vi "Window-Functional data editor - variable patch.vi"(9 "Experiment Path":path=path "D:/Microscope data/Sameer/2019-10-16/191016_19_21_07 FunctAcq", 11 "Standalone viewer?":bool=TRUE) -> ()   [LabVIEW 2020]
uses:
  User Interface/Visualisation/Timelapse Viewer/Typedefs/Custom slider-vertical.ctl
  User Interface/Visualisation/Timelapse Viewer/Typedefs/Colour.ctl
  User Interface/Visualisation/Timelapse Viewer/Typedefs/Channel to load.ctl
  User Interface/Visualisation/Timelapse Viewer/Typedefs/Time series viewer refs.ctl
  User Interface/Visualisation/Timelapse Viewer/Typedefs/Speed Viewer States enum.ctl
  <vilib>/Utility/miscctls.llb/LVPointTypeDef.ctl
  <vilib>/vision/Image Controls.llb/IMAQ Image.ctl
  Typedefs/HW config states enum.ctl
  User Interface/Visualisation/Functional Imaging Viewer/Typedefs/Get-Set-Clear Control.ctl
  User Interface/Visualisation/Timelapse Viewer/Typedefs/Select Play-Stop button to show.ctl
  <vilib>/Utility/error.llb/DialogType.ctl
  User Interface/Visualisation/Timelapse Viewer/Cam video sync/Typedefs/Cam videos cluster.ctl
  User Interface/Visualisation/Timelapse Viewer/Globals/gl_Time series viewer globals.vi
  Global Variables/General Globals.vi
  Typedefs/Save-Load enum.ctl
panel:
  in  "Image Scrollbar":i32(c297)
  out "VL Image Array":T1[](array[plugin-control])
  in  "Channel to load":T2
  in  "Number of rows to generate":i32=3 format="%.0f rows"
  in  "Source number of frames":T3(ring)=enum."As many as the number of cycles"
  out "Slider at frame #":i32 format="Cycle %.0f"
  in  "Scrollbar":i32(c297)
  in  "Back":bool
  in  "Play":bool
  in  "Stop":bool
  in  "Tab Control":enum32{"Camera videos", "Speed data"}(tab)
  out "Cams":T4 {"Vid4 Rel time (ms)" format="%.0f ms"; "Vid3 Rel time (ms)" format="%.0f ms"; "Vid2 Rel time (ms)" format="%.0f ms"; "Vid1 Rel time (ms)" format="%.0f ms"}
  out "Actual number \nof speed points":i32 format="Actual of speed points: %.0f"
  out "Speed Data":string[][](array[string])
  out "Expected speed values":dbl format="Expected speed points: %#_g"
  out "Original frame rate (fps)":dbl format="Original frame rate: %#.1f (fps)"
  out "Frame rate set (fps)":dbl format="Frame rate set: %#.1f (fps)"
  out "Actual frame rate (fps)":dbl format="Actual frame rate: %#.1f (fps)"
  out "AVI Mode ind":string="AVI mode:"
  out "Video length info":string="Duration: 00h 00m 00s, 0 frames"
  out "Export images":bool
  out "Export snippet":bool
  in  "Extraction Cursors":cluster{i32, i32}(slide)={1, 5594} scale=1.0..1109.0
  out "Export vid":bool
  out "Stop (ind)":bool
  in  "Intensity":T5={0.0, 4095.0} scale=0.0..4095.0
  in  "Colour":T6
  out "Speed Graph":dbl[](graph) caption="Speed Chart"
  out "Image":T1(plugin-control)
  # "Date                         Time                  Time stamp           Speed (rpm)          Angle (deg)"
  # "Timelapse Info"
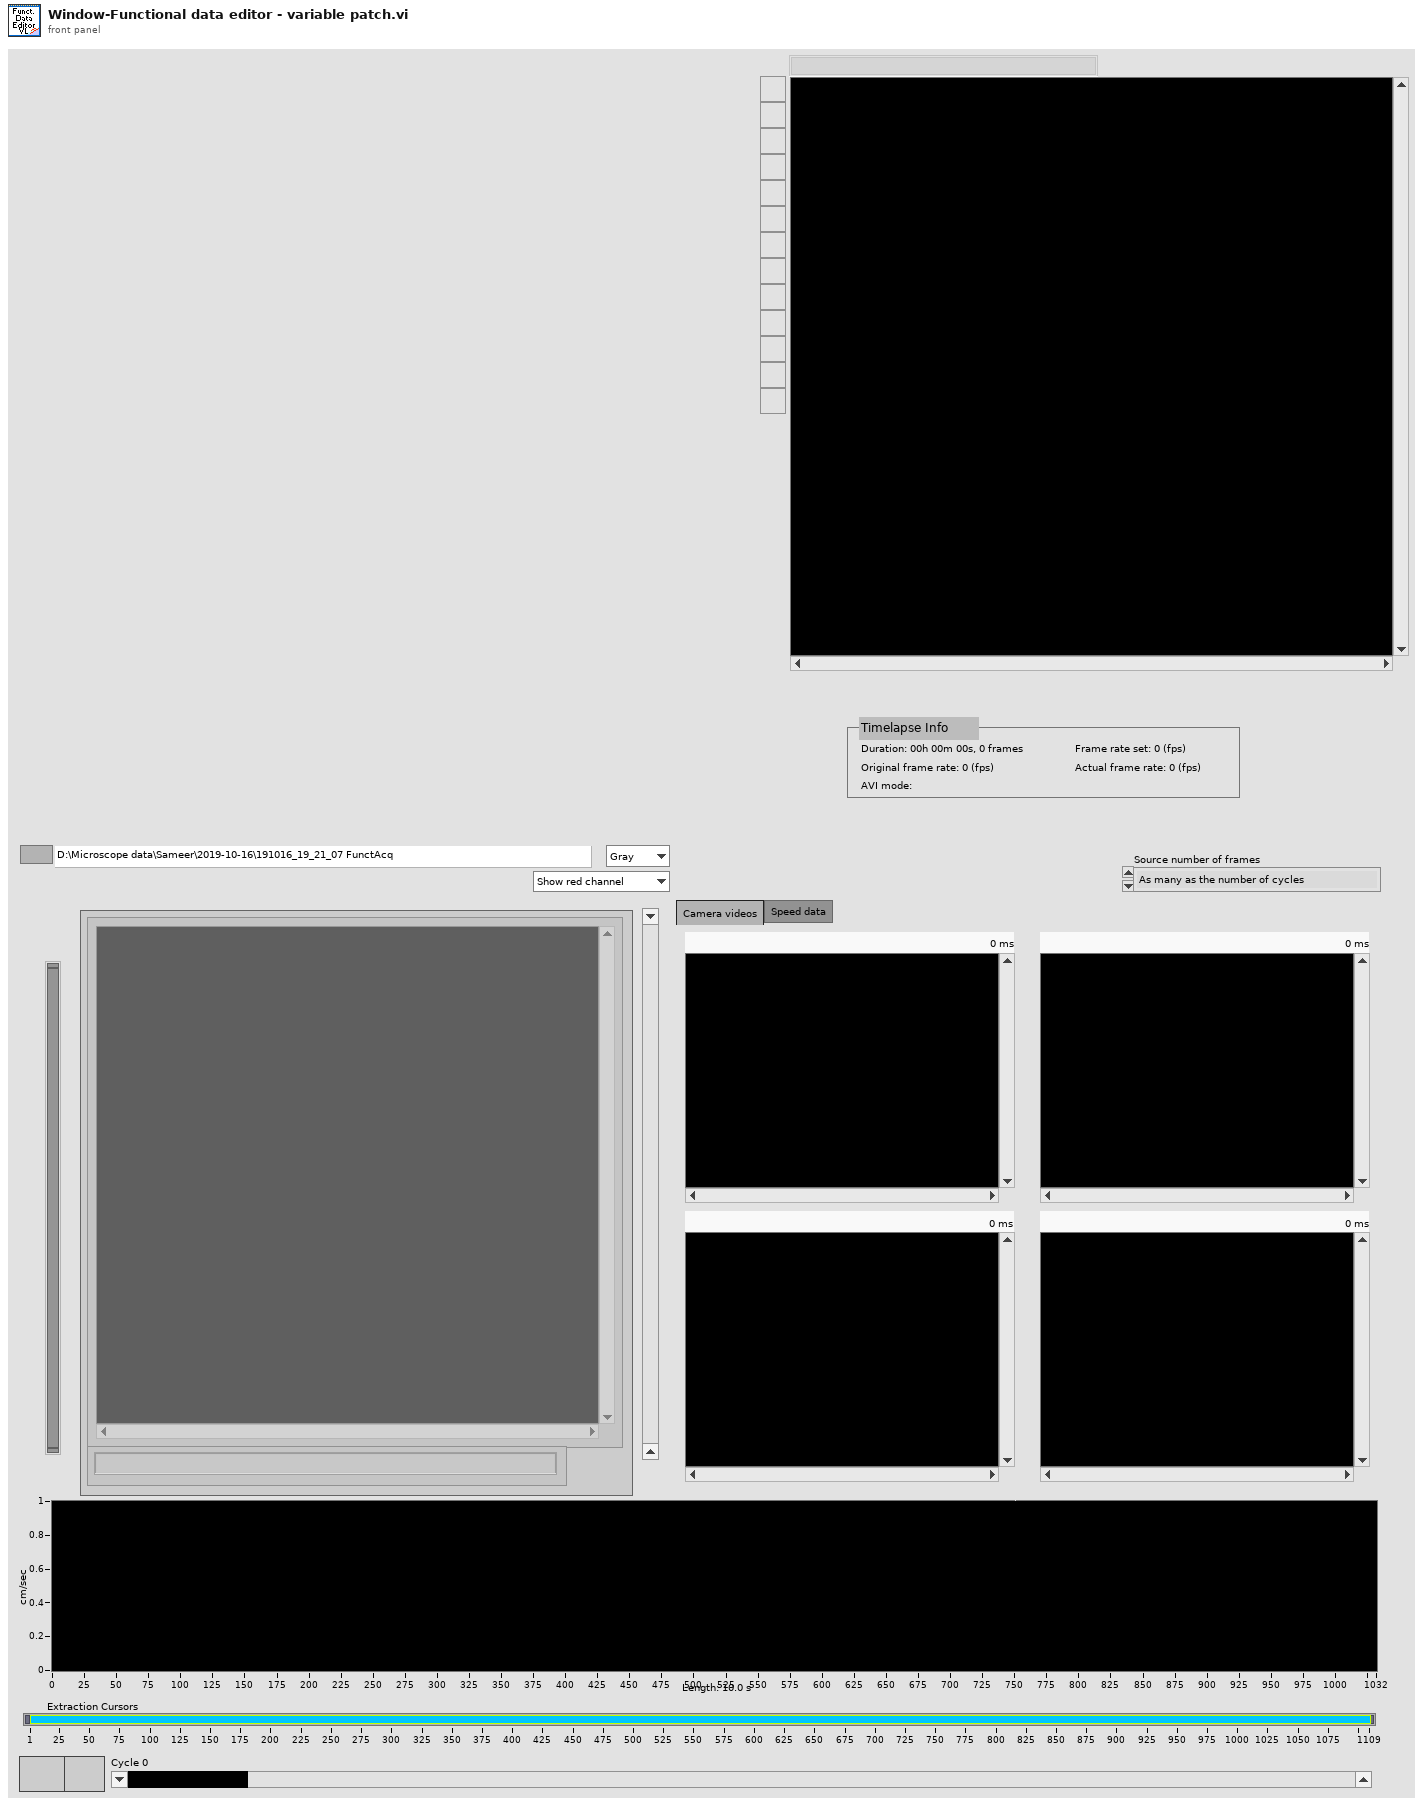
[diagram p1: front panel]
types:
  T1 = typedef "IMAQ Image.ctl" = refnum<image>
  T2 = typedef "Channel to load.ctl" = enum16{"Show red channel", "Show green channel", "Show both channels"}
  T3 = enum16{"As many as the frames in the video with the fewest frames", "As many as the number of cycles"}
  T4 = cluster{"Vid 1":T1, "Vid 2":T1, "Vid 3":T1, "Vid 4":T1, "Vid1 Rel time (ms)":u32, "Vid2 Rel time (ms)":u32, "Vid3 Rel time (ms)":u32, "Vid4 Rel time (ms)":u32}
  T5 = typedef "Custom slider-vertical.ctl" = cluster{dbl, dbl}
  T6 = typedef "Colour.ctl" = enum16{"Gray", "Red", "Green", "Mixed"}
  T7 = typedef "Time series viewer refs.ctl" = cluster{"This VI":refnum<vi>, "Image control":refnum<vi>, "AVI Mode ind":refnum<vi>, "Play":refnum<vi>, "Stop":refnum<vi>, "Back":refnum<vi>, "Scrollbar":refnum<vi>, "Video length info":refnum<vi>, "Expected speed values":refnum<vi>, "Intensity":refnum<vi>, "Path":refnum<vi>, "Selection sliders":refnum<vi>, "Speed Graph ref":refnum<vi>, "Frame rate set (fps)":refnum<vi>, "Number of rows to generate":refnum<vi>, "VL Image Array":refnum<vi>, "Image Scrollbar":refnum<vi>, "Channel to load":refnum<vi>, "Colour":refnum<vi>}
  T8 = enum16{"None", "Release queue", "Obtain queue", "Enqueue", "Get status", "Set status"}
  T9 = typedef "LVPointTypeDef.ctl" = cluster{"Horizontal":i16, "Vertical":i16}
  T10 = typedef "Speed Viewer States enum.ctl" = enum16{"Idle", "Initialise", "Playback", "Scroll bar event", "Speed cursor event", "Back to start", "Exit"}
  T11 = typedef "Save-Load enum.ctl" = enum16{"Save to file", "Load from file", "Compare from file", "Save Backup"}
  T12 = typedef "HW config states enum.ctl" = enum16{"Load from file", "Save to file", "Save backup", "Write all", "Read all", "Write XY stage settings", "Write DAQ FPGA settings", "Write Control FPGA settings", "Write Phys Channels", "Write System Config", "Write HW Config", "Save System Config", "Save HW Config", "Clear", "Compare from file"}
  T13 = typedef "Image Type" = u32
  T14 = typedef "Custom slider-horisontal.ctl" = cluster{dbl, dbl}
  T15 = typedef "Cam videos cluster.ctl" = cluster{"Vid 1":T1, "Vid 2":T1, "Vid 3":T1, "Vid 4":T1, "Vid1 Rel time (ms)":u32, "Vid2 Rel time (ms)":u32, "Vid3 Rel time (ms)":u32, "Vid4 Rel time (ms)":u32}
  T16 = typedef "Get-Set-Clear Control.ctl" = enum16{"Get", "Set", "Clear"}
  T17 = typedef "Select Play-Stop button to show.ctl" = enum16{"Show Play button", "Show Stop button"}
  T18 = typedef "DialogType.ctl" = u16
  T19 = typedef "Hardware Configuration settings.ctl" = cluster{"Dev. PC":bool, "Swap XY on stage":bool, "No of AOD":u8, "MC Supported":bool, "Axial MC":bool, "Computer MAC address":string, "Externalise Triggers":bool, "Trigger HW config":T20, "DAQmx Chan":T21, "XYZ Stage Control Config":T22, "XY stage available":bool, "XY Comms Config Cluster":T23, "Y stage available":bool, "Y Comms Config Cluster":T23, "Z stage available":bool, "Z Comms Config Cluster ":T23, "Encoder available":bool, "Encoder":T25, "VidRec available":bool, "Cam VidRec":T26, "Laser Power Control HW config":T27, "Laser 1 available":bool, "Laser 1 config cluster":T28, "Prechirper 1 available":bool, "Prechirper 1 config cluster":T29, "Control system.FPGA available?":bool, "Control Sys. HW config":T30, "DAQ FPGA HW Config":T31, "PMT Control Voltage Limits":T35}
  T20 = typedef "Triggers HW config.ctl" = cluster{"Available Device List":i32, "Device Address":string}
  T21 = typedef "DAQmx physical channels cluster.ctl" = cluster{"Pockels AO":tag, "Hard shutter AO":tag, "PMT AOs":tag, "Galvo AOs":tag, "Power meter AI":tag}
  T22 = typedef "XYZControlConfig.ctl" = enum16{"None", "XYZ", "XY-Z", "X-Y-Z", "Z"}
  T23 = typedef "Peripherals comms config cluster.ctl" = cluster{"Name":string, "Device Address":string, "Port ":u16, "Baudrate":i32, "Comms Type":T24}
  T24 = typedef "Comms Type.ctl" = enum16{"GPIB-IEEE488", "Serial-RS232", "Serial-RS485", "Serial-RS422", "Serial-USB", "Ethernet-TCP/IP", "Ethernet-UDP"}
  T25 = typedef "Encoder config cluster.ctl" = cluster{"IP address":string, "Port":u16, "Wheel radius (cm)":dbl, "Encoder Trigger":tag}
  T26 = typedef "Cam VidRec HW config setup cluster.ctl" = cluster{"DO flag-Video record":tag, "DO flag-Trial start":tag}
  T27 = typedef "Laser Power Control HW config.ctl" = cluster{"Laser Power Control":string, "Laser Power Modulation Control":enum16{"NI", "FPGA"}}
  T28 = typedef "Laser 1 config cluster.ctl" = cluster{"COM port":refnum<visa-resource-name>, "Baud Rate":i32, "Type":string}
  T29 = typedef "PreChirper 1 config cluster.ctl" = cluster{"Type":string, "Baud Rate":i32, "COM port":refnum<visa-resource-name>}
  T30 = typedef "Control Sys HW config cluster.ctl" = cluster{"Control system.FPGA Type":enum16{"Virtex 5", "Virtex 7"}, "Control system.Network adapter name":string, "Control system.MAC address":string, "Control system.Ethernet Port":u32, "Control system.Ethernet Port Opened":bool}
  T31 = typedef "DAQ FPGA HW config cluster.ctl" = cluster{"FGPA Ref":T32, "Target":T33, "input card type":T34}
  T32 = typedef "FPGA Ref.ctl" = refnum<k20>
  T33 = typedef "nirio_resource_hc.ctl" = tag
  T34 = typedef "FPGA input type AC-DC.ctl" = enum16{"AC Card", "DC Card"}
  T35 = typedef "PMT Control Voltage limits.ctl" = cluster{"Lower Limit":dbl, "Upper Limit":dbl}
  T36 = cluster{"Start Frame No":i32, "End Frame No":i32}
  T37 = typedef "IMAQ AVI2 Refnum.ctl" = refnum<k20>
  T38 = cluster{"# of frames to export":i32, "Initial frame's owning file":T37, "8-bit AVI file path":path, "Cursors location":cluster{"Number of first frame":i32, "Number of last frame":i32}}
  T39 = enum32{"Invalid", "Standard", "Closed", "Hidden", "Minimized", "Maximized"}
  T40 = typedef "Speed graph behaviour enum.ctl" = enum16{"Scrolling data", "Scrolling cursor"}
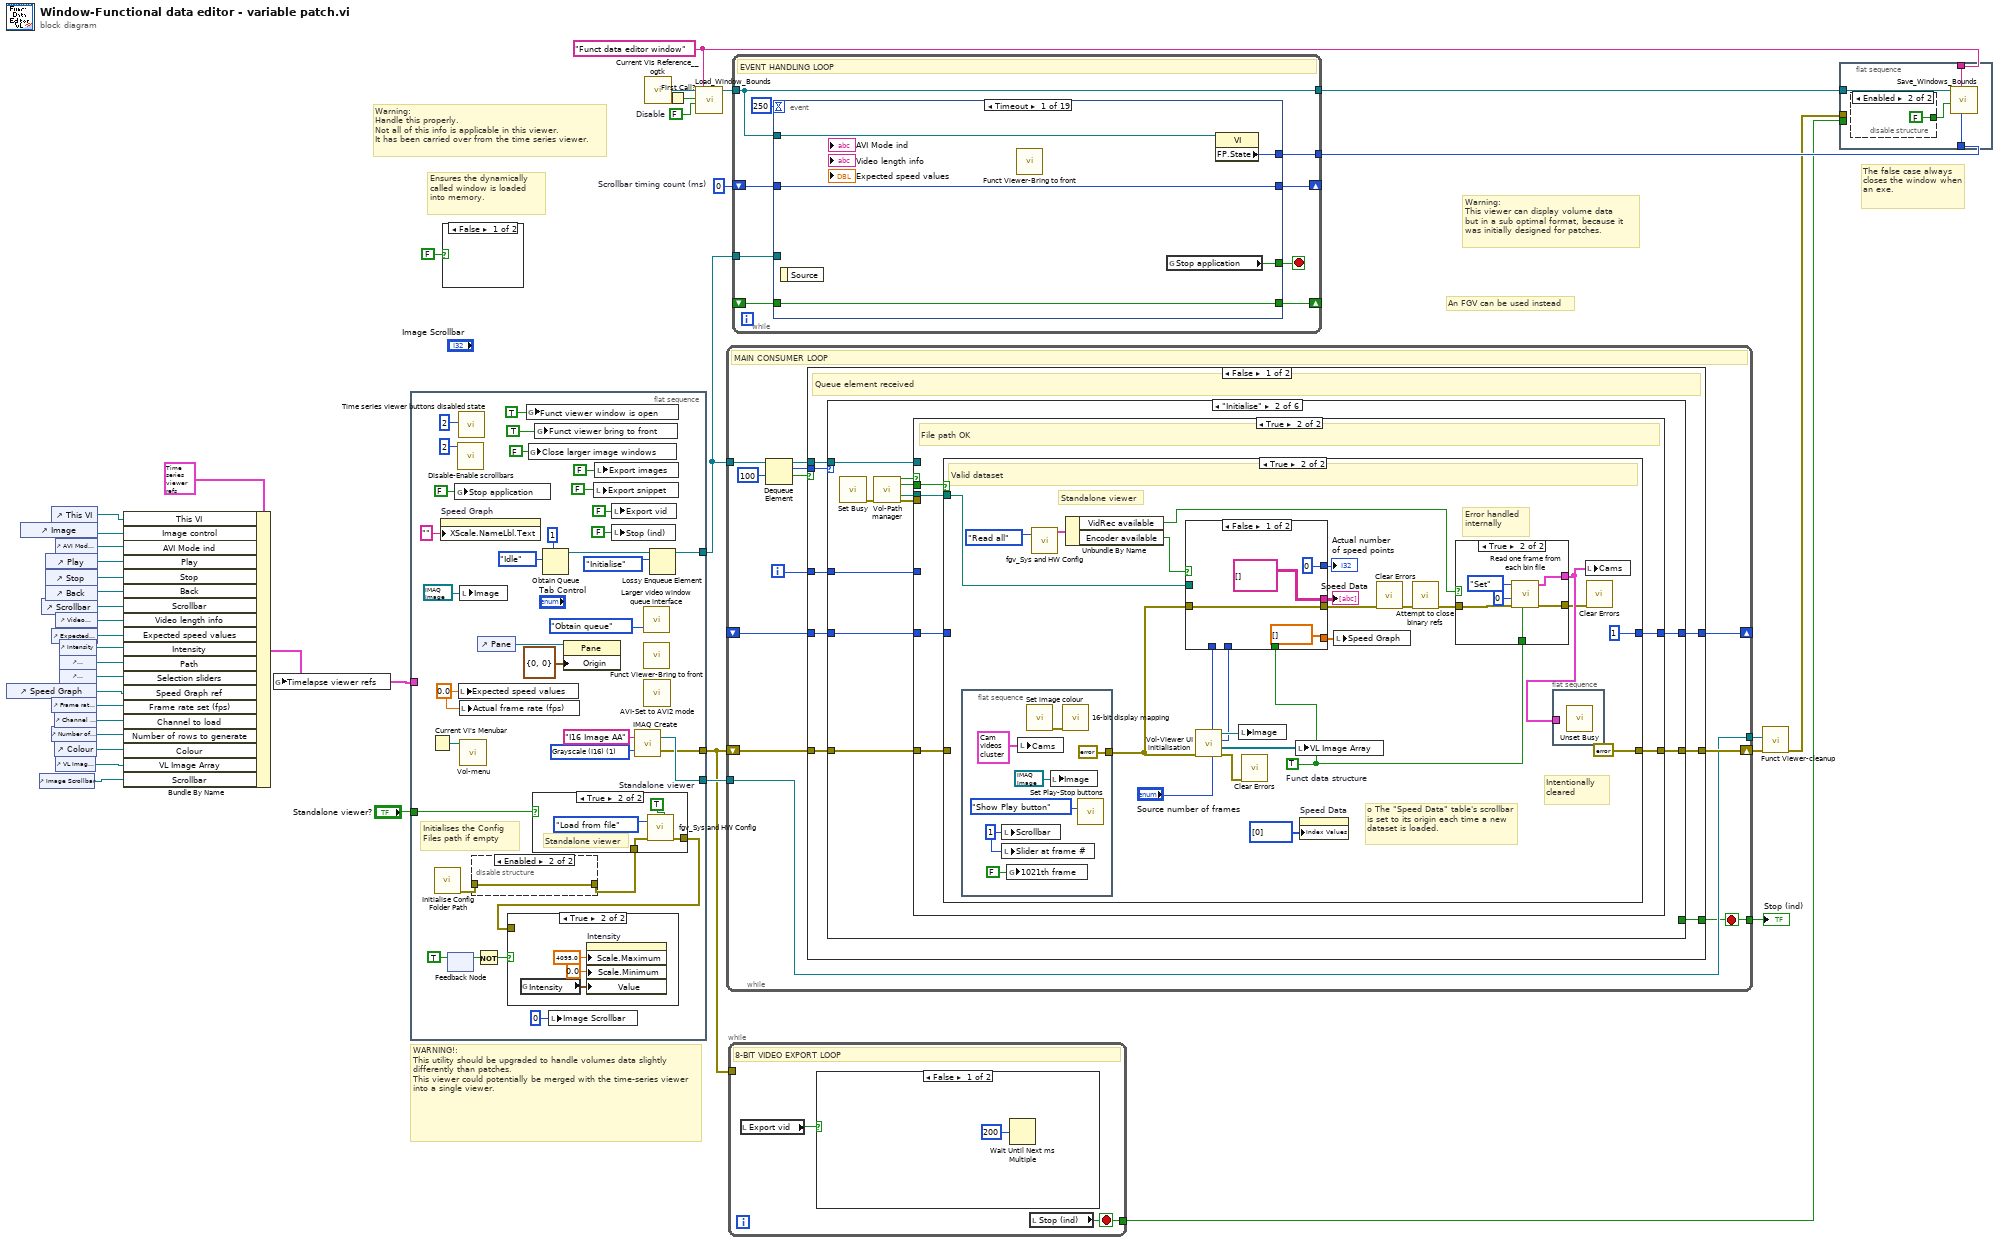
[diagram p0: block diagram]
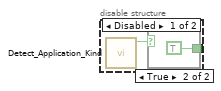
[diagram p2: hidden frame]
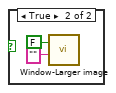
[diagram p4: hidden frame]
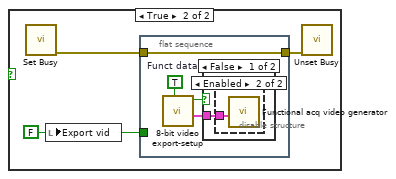
[diagram p5: hidden frame]
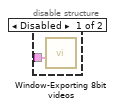
[diagram p6: hidden frame]
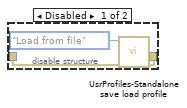
[diagram p8: hidden frame]
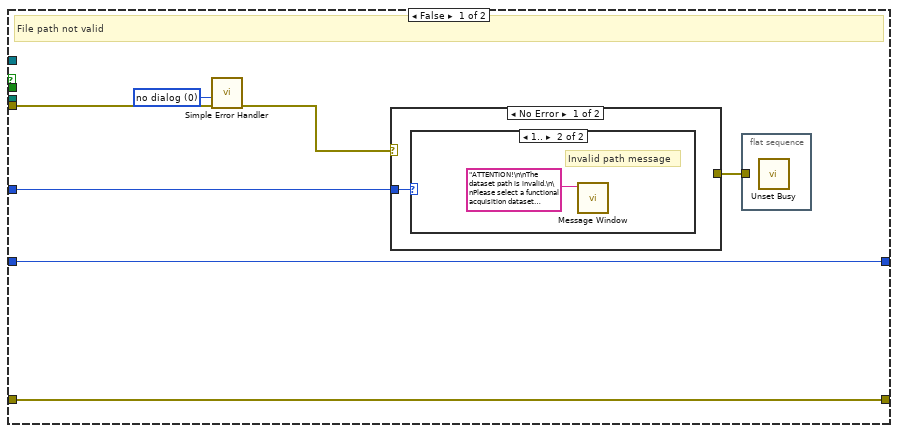
[diagram p12: hidden frame]
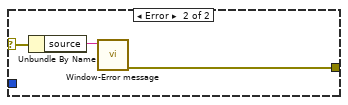
[diagram p14: hidden frame]
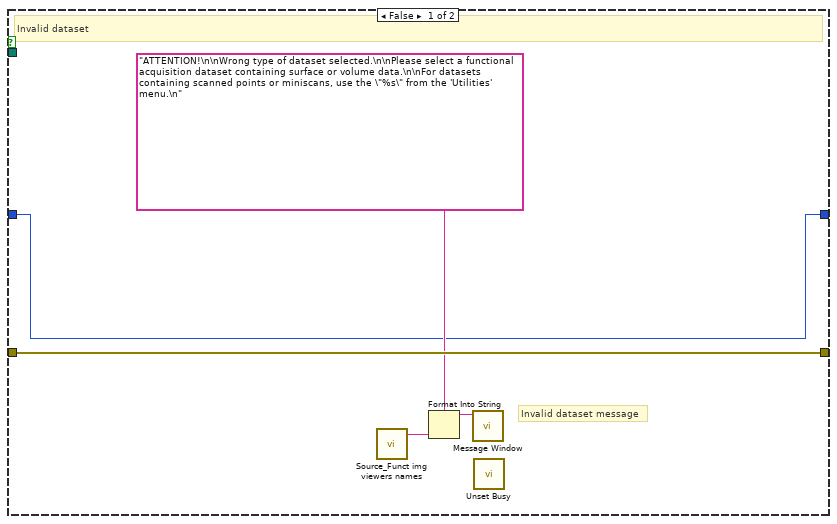
[diagram p15: hidden frame]
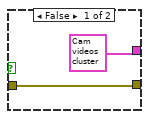
[diagram p16: hidden frame]
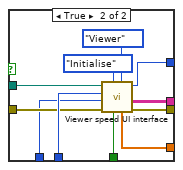
[diagram p17: hidden frame]
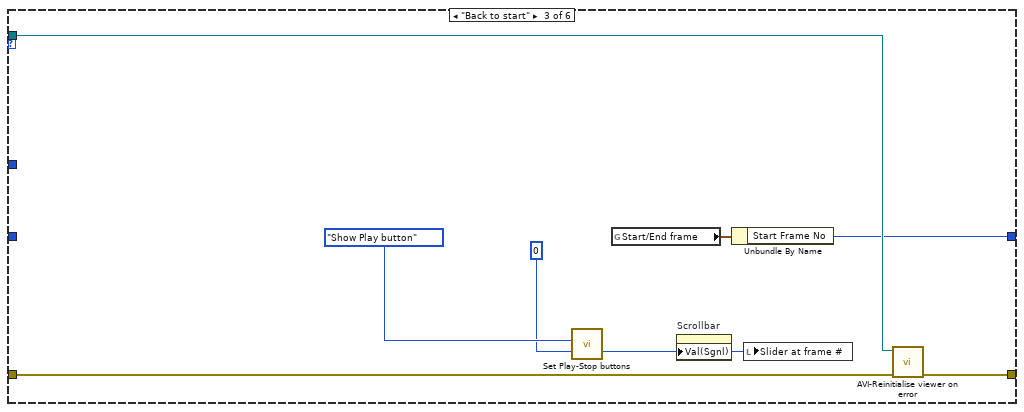
[diagram p18: hidden frame]
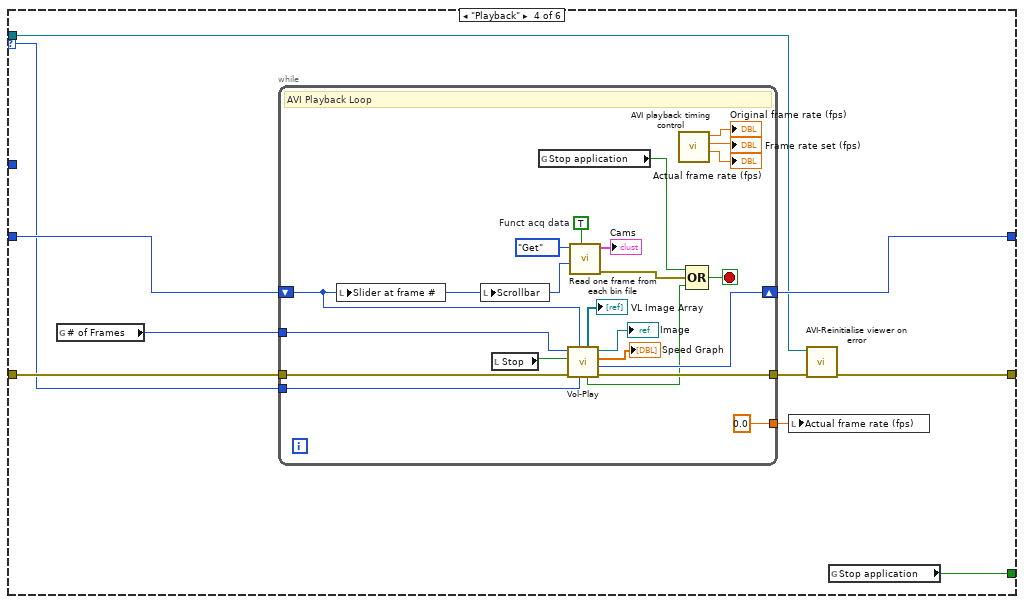
[diagram p19: hidden frame]
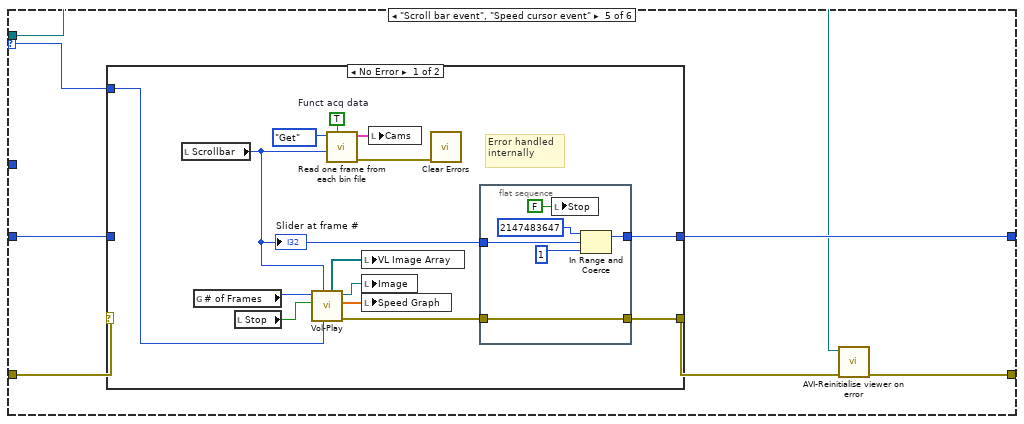
[diagram p20: hidden frame]
diagram:
  w17 = FALSE  # Disable
  w16 = "Funct data editor window" ("Window Name (i.e. Key)")
  w26 = u32 0  # Scrollbar timing count (ms)
  # "Warning:\nThis viewer can display volume data\nbut in a sub optimal format, because it\nwas initially designed for patches."
  # "Warning:\nHandle this properly.\nNot all of this info is applicable in this viewer.\nIt has been carried over from the time series viewer."
  # "WARNING!:\nThis utility should be upgraded to handle volumes data slightly differently than patches.\nThis viewer could potentially be merged with the time-series viewer into a single viewer."
  # "The false case always closes the window when an exe."
  # "Ensures the dynamically called window is loaded into memory."
  # "An FGV can be used instead"
  n1 = control-ref of="Speed Graph"() -> (w21:refnum<vi>)
  n2 = control-ref of="Image"() -> (w6:refnum<vi>)
  n3 = control-ref of="Image Scrollbar"() -> (w3:refnum<vi>)
  n4 = control-ref of="Scrollbar"() -> (w30:refnum<vi>)
  n5 = control-ref of="Play"() -> (w33:refnum<vi>)
  n6 = control-ref of="Stop"() -> (w32:refnum<vi>)
  n7 = control-ref of="Back"() -> (w31:refnum<vi>)
  n8 = control-ref of="Frame rate set (fps)"() -> (w10:refnum<vi>)
  n9 = control-ref of="Number of rows to generate"() -> (w8:refnum<vi>)
  n10 = control-ref of="This VI"() -> (w24:refnum<vi>)
  n11 = control-ref of="Expected speed values"() -> (w28:refnum<vi>)
  n12 = control-ref of="Channel to load"() -> (w1:refnum<vi>)
  n13 = control-ref of="Colour"() -> (w2:refnum<vi>)
  n14 = control-ref of="AVI Mode ind"() -> (w36:refnum<vi>)
  n15 = control-ref of="Video length info"() -> (w29:refnum<vi>)
  n16 = control-ref of="VL Image Array"() -> (w4:refnum<vi>)
  n17 = control-ref of="Intensity"() -> (w27:refnum<vi>)
  n18 = control-ref of="Experiment Path"() -> (w25:refnum<vi>)
  n19 = control-ref of="Extraction Cursors"() -> (w22:refnum<vi>)
  n20 = Bundle By Name(cluster=T7 {"This VI"=refnum, "Image control"=refnum, "AVI Mode ind"=refnum, "Play"=refnum, "Stop"=refnum, "Back"=refnum, "Scrollbar"=refnum, "Video length info"=refnum, "Expected speed values"=refnum, "Intensity"=refnum, "Path"=refnum, "Selection sliders"=refnum, "Speed Graph ref"=refnum, "Frame rate set (fps)"=refnum, "Number of rows to generate"=refnum, "VL Image Array"=refnum, "Image Scrollbar"=refnum, "Channel to load"=refnum, "Colour"=refnum}, "This VI"=w24, "Image control"=w6, "AVI Mode ind"=w36, "Play"=w33, "Stop"=w32, "Back"=w31, "Scrollbar"=w30, "Video length info"=w29, "Expected speed values"=w28, "Intensity"=w27, "Path"=w25, "Selection sliders"=w22, "Speed Graph ref"=w21, "Frame rate set (fps)"=w10, "Channel to load"=w1, "Number of rows to generate"=w8, "Colour"=w2, "VL Image Array"=w4, "Scrollbar"=w3) -> (w5:T7)
  n21 = global write "gl_Time series viewer globals.vi" "Timelapse viewer refs"(w5) -> ()
  n22 = flat-sequence {
    tunnel: [w71] -> w39
    tunnel: [w45] -> w20
    tunnel: [w68] -> w37
    tunnel: w5 -> [_]
    tunnel: "Standalone viewer?" -> [w44]
    frame #0 {
      w64 = 0.0 ("Expected speed points")
      w73 = T13 1 items=["Grayscale (U8)", "Grayscale (I16)", "Grayscale (SGL)", "Complex (CSG)", "RGB (U32)", "HSL (U32)", "RGB (U64)", "Grayscale (U16)"] ("Image Type")
      # "Initialises the Config Files path if empty"
      n23 = Current VI's Menubar() -> (w63:refnum<k9>)
      n24 = call "Initialise Config Folder Path.vi"() -> ("error out"=w50:errorcluster)  [unwired: 9 in, 2 out]
      n25 = property on="Speed Graph" class="WFGraph (strict)"("XScale.NameLbl.Text"="" ("X Scale.Name Label.Text")) -> ()  [unwired: 2 in, 2 out]
      n26 = feedback #1() -> (w46:bool)  [unwired: 1 in]
      n27 = feedback-in #1(TRUE) -> ()
      n28 = global write "General Globals.vi" "Stop application"(FALSE ("Stop application")) -> ()
      n29 = call "Disable-Enable scrollbars.vi"("Disabled state"=2) -> ()  [unwired: 10 in, 1 out]
      n30 = call "Time series viewer buttons disabled state.vi"("Disabled"=2) -> ()  [unwired: 10 in, 1 out]
      n31 = local write "Expected speed values"(w64) -> ()
      n32 = local write "Actual frame rate (fps)"(w64) -> ()
      n33 = local write "Image"(T1 refnum ("Image")) -> ()
      n34 = call "Vol-menu.vi"("menu"=w63) -> ()  [unwired: 9 in, 2 out]
      n35 = disable-structure shown="Enabled" {
        disable-tunnel: w50 -> [w75 w77]
        disable-tunnel: [w74 w77] -> w43
        frame Disabled {
          n36 = call "UsrProfiles-Standalone save load profile.vi"("Error in"=w75, "Function"=Save-Load_enum."Load from file") -> ("error out"=w74:errorcluster)  [unwired: 9 in]
        }
        frame Enabled {
        }
      }
      n37 = Not(x=w46) -> (.not. x?=w48:bool)
      n38 = control-ref of="Pane"() -> (w65:refnum<vi>)
      n39 = global write "gl_Time series viewer globals.vi" "Funct viewer window is open"(TRUE ("Bring Timelapse Editor to front")) -> ()
      n40 = global write "gl_Time series viewer globals.vi" "Close larger image windows"(FALSE ("Close larger image window")) -> ()
      n41 = case shown="True" w44 {
        tunnel: w43 -> [w78 w81]
        tunnel: [w78 w80] -> w42
        frame False {
          # "No need to load the system\nconfig. Already loaded."
        }
        frame True {
          w79 = TRUE  # Standalone viewer
          # "Standalone viewer"
          n42 = call "fgv_Sys and HW Config.vi"("Standalone viewer initialisation?"=w79, "Function"=HW_config_states_enum."Load from file", "error in (no error)"=w81) -> ("error out"=w80:errorcluster)  [unwired: 6 in, 2 out]
        }
      }
      n43 = case shown="True" w48 {
        tunnel: w42 -> [_ _]
        frame False {
        }
        frame True {
          n44 = global read "gl_Time series viewer globals.vi" "Intensity"() -> (w83:T14)
          n45 = property on="Intensity" class="Slide (strict)"("Scale.Maximum"=4095.0 ("Scale.Range:Maximum"), "Scale.Minimum"=0.0 ("Scale.Range:Minimum"), "Value"=w83) -> ()  [unwired: 2 in, 2 out]
        }
      }
      n46 = global write "gl_Time series viewer globals.vi" "Funct viewer bring to front"(TRUE ("Window is open")) -> ()
      n47 = Obtain Queue(max queue size (-1, unlimited)=1, element data type=Speed_Viewer_States_enum."Idle" ("States")) -> (queue out=w69:refnum<queue>)  [unwired: 3 in, 2 out]
      n48 = local write "Image Scrollbar"(0 ("Image Scrollbar")) -> ()
      n49 = property class="Pane"(reference=w65, "Origin"=T9 {"Horizontal"=0, "Vertical"=0}) -> ()  [unwired: 1 in, 2 out]
      n50 = local write "Export snippet"(FALSE ("Export data subset")) -> ()
      n51 = local write "Export images"(FALSE ("Export data subset")) -> ()
      n52 = local write "Export vid"(FALSE ("Export")) -> ()
      n53 = local write "Stop (ind)"(FALSE ("Boolean")) -> ()
      n54 = call "IMAQ Create"("Image Name"="I16 Image AA", "Image Type"=w73) -> ("New Image"=w71:T1, "error out"=w45:errorcluster)  [unwired: 2 in, 1 out]
      n55 = call "Larger video window queue interface.vi"("Function"=T8."Obtain queue") -> ()  [unwired: 10 in, 1 out]
      n56 = call "Funct Viewer-Bring to front.vi"() -> ()  [unwired: 12 in]
      n57 = call "AVI-Set to AVI2 mode.vi"() -> ()  [unwired: 11 in, 1 out]
      n58 = Lossy Enqueue Element(queue=w69, element=Speed_Viewer_States_enum."Initialise" ("States")) -> (queue out=w68:refnum<queue>)  [unwired: 1 in, 3 out]
    }
  }
  n59 = case shown="False" FALSE {
    frame False {
    }
    frame True {
      n60 = call "Window-Larger image.vi"("Image name"="", "Open maximised"=FALSE) -> ()  [unwired: 10 in]
    }
  }
  n61 = call <userlib>:"Current VIs Reference__ogtk.vi"() -> ("Current VI's reference"=w19:refnum<vi>)  [unwired: 5 in]
  n62 = First Call?() -> (First Call?: T/F=w18:bool)
  n63 = call "Load_Window_Bounds.vi"("Window Name (i.e. Key)"=w16, "Disable"=w17, "First Call"=w18, "Window VI's Ref"=w19) -> ("reference out"=w13:refnum<vi>)  [unwired: 4 in, 3 out]
  n64 = while {
    tunnel: w39 -> [w91]
    tunnel: [w91] -> w38
    shift-right: [w97] -> _
    shift-left: _ -> [w96]
    tunnel: w37 -> [w95]
    shift-right: [w98] -> w34
    shift-left: w20 -> [w99]
    tunnel: [w90] -> w23
    i -> [w89]
    stop <- w90 stop-if-true
    # "MAIN CONSUMER LOOP"
    n65 = Dequeue Element(queue=w95, timeout in ms (-1)=100) -> (queue out=w88:refnum<queue>, element=w92:T10, timed out?=w93:bool)  [unwired: 1 in, 1 out]
    n66 = case shown="False" w93 {
      tunnel: w99 -> [w107 w271]
      tunnel: [w106 w271] -> w98
      tunnel: [w105 w272] -> w97
      tunnel: w96 -> [w104 w272]
      tunnel: w92 -> [w103 _]
      tunnel: [w102 w270] -> w90
      tunnel: w88 -> [w101 _]
      tunnel: w89 -> [w100 _]
      frame False {
        # "Queue element received"
        n67 = case shown="\"Initialise\"" w103 {
          selector: w103 -> [_ _ _ w205 w236 _]
          tunnel: w107 -> [w108 w119 w203 w214 w241 w265]
          tunnel: [w108 w118 w202 w211 w239 w265] -> w106
          tunnel: [w109 w120 w199 w213 w242 1 ("Slide")] -> w105
          tunnel: w104 -> [w109 w117 _ w212 w240 _]
          tunnel: [_ _ _ w206 _ TRUE] -> w102
          tunnel: w101 -> [_ w116 w201 w209 w237 _]
          tunnel: w100 -> [_ w115 _ _ _ _]
          frame Default {
          }
          frame "Initialise" {
            n68 = call <vilib>:"Set Busy.vi"() -> ("error out"=w111:errorcluster)  [unwired: 10 in, 1 out]
            n69 = call "Vol-Path manager.vi"("error in (no error)"=w111) -> ("File path OK"=w114:bool, "Valid data type (& valid path)"=w110:bool, "Speed Data folder path+dummy filename"=w113:path, "error"=w112:errorcluster)  [unwired: 10 in, 1 out]
            n70 = case shown="True" w114 {
              tunnel: [w127 w136] -> w120
              tunnel: w113 -> [_ w137]
              tunnel: w119 -> [w126 w133]
              tunnel: [w126 w138] -> w118
              tunnel: w117 -> [w127 w134]
              tunnel: w112 -> [w125 _]
              tunnel: w116 -> [_ _]
              tunnel: w115 -> [w122 _]
              tunnel: w110 -> [_ w135]
              frame False {
                w124 = T18 0 items=["no dialog", "OK message", "continue or stop message", "OK message + warnings", "continue/stop + warnings"] ("type of dialog (OK msg:1)")
                # "File path not valid"
                n71 = call <vilib>:"Simple Error Handler.vi"("type of dialog (OK msg:1)"=w124, "error in (no error)"=w125) -> ("error out"=w123:errorcluster)  [unwired: 3 in, 4 out]
                n72 = case shown="No Error" w123 {
                  selector: w123 -> [_ w132]
                  tunnel: w122 -> [w128 _]
                  tunnel: [_ w130] -> w121
                  frame No Error {
                    n73 = case shown="1.." w128 {
                      frame 0, Default {
                      }
                      frame 1.. {
                        # "Invalid path message"
                        n74 = call "Message Window.vi"("Message string"="ATTENTION!\n\nThe dataset path is invalid.\n\nPlease select a functional acquisition dataset containing surface or volume data.\n") -> ()  [unwired: 10 in, 1 out]
                      }
                    }
                  }
                  frame Error {
                    n75 = Unbundle By Name(w132) -> ("source"=w131:string)
                    n76 = call "Window-Error message.vi"("Message"=w131) -> ("Error Out (no error)"=w130:errorcluster)  [unwired: 10 in]
                  }
                }
                n77 = flat-sequence {
                  tunnel: w121 -> [_]
                  frame #0 {
                    n78 = call <vilib>:"Unset Busy.vi"() -> ()  [unwired: 11 in, 1 out]
                  }
                }
              }
              frame True {
                # "File path OK"
                n79 = case shown="True" w135 {
                  tunnel: [w143 errorcluster {"status"=FALSE, "code"=0, "source"=""} ("error out")] -> w138
                  tunnel: w137 -> [_ w166]
                  tunnel: [w140 1 ("Slide")] -> w136
                  tunnel: w134 -> [w140 _]
                  tunnel: w133 -> [w143 _]
                  frame False {
                    # "Invalid dataset message"
                    # "Invalid dataset"
                    n80 = call "Source_Funct img viewers names.vi"() -> ("Name string: Functional imaging viewer (POI/Mscn)"=w141:string)  [unwired: 10 in, 1 out]
                    n81 = Format Into String(format string="ATTENTION!\n\nWrong type of dataset selected.\n\nPlease select a functional acquisition dataset containing surface or volume data.\n\nFor datasets containing scanned points or miniscans, use the \"%s\" from the 'Utilities' menu.\n" ("Message"), w141) -> (resulting string=w139:string)  [unwired: 2 in, 1 out]
                    n82 = call "Message Window.vi"("Message string"=w139) -> ()  [unwired: 10 in, 1 out]
                    n83 = call <vilib>:"Unset Busy.vi"() -> ()  [unwired: 11 in, 1 out]
                  }
                  frame True {
                    w150 = TRUE  # Funct data structure
                    # "Standalone viewer"
                    # "o\tThe \"Speed Data\" table's scrollbar is set to its origin each time a new dataset is loaded."
                    # "Error handled internally"
                    # "Intentionally cleared"
                    # "Valid dataset"
                    n84 = flat-sequence {
                      tunnel: [errorcluster {"status"=FALSE, "code"=0, "source"=""} ("error out")] -> w157
                      frame #0 {
                        w192 = 1 ("Scrollbar")
                        n85 = local write "Scrollbar"(w192) -> ()
                        n86 = local write "Slider at frame #"(w192) -> ()
                        n87 = global write "gl_Time series viewer globals.vi" "1021th frame"(FALSE ("1021th frame")) -> ()
                        n88 = local write "Cams"(T15 {"Vid 1"=refnum, "Vid 2"=refnum, "Vid 3"=refnum, "Vid 4"=refnum, "Vid1 Rel time (ms)"=0, "Vid2 Rel time (ms)"=0, "Vid3 Rel time (ms)"=0, "Vid4 Rel time (ms)"=0} ("Cam videos cluster")) -> ()
                        n89 = call "Set image colour.vi"() -> ("error out"=w191:errorcluster)  [unwired: 11 in]
                        n90 = local write "Image"(T1 refnum ("New Image")) -> ()
                        n91 = call "16-bit display mapping.vi"("error in (no error)"=w191) -> ()  [unwired: 10 in, 1 out]
                        n92 = call "Set Play-Stop buttons.vi"("Function"=Select_Play-Stop_button_to_show."Show Play button") -> ()  [unwired: 10 in, 1 out]
                      }
                    }
                    n93 = call "fgv_Sys and HW Config.vi"("Function"=HW_config_states_enum."Read all") -> ("Hardware Configuration OUT"=w147:T19)  [unwired: 8 in, 2 out]
                    n94 = Unbundle By Name(w147) -> ("VidRec available"=w145:bool, "Encoder available"=w146:bool)
                    n95 = call "Vol-Viewer UI initialisation.vi"("Source number of frames"="Source number of frames", "error in (no error)"=w157) -> ("error out"=w152:errorcluster, "VL array refs"=w144:T1[], "Number of Frames"=w162:u32, "Image ref"=w163:T1, "Scrollbar position"=w151:i32)  [unwired: 5 in]
                    n96 = case shown="False" w146 {
                      tunnel: w166 -> [_ w190]
                      tunnel: [dbl[] [] ("Speed waveform graph data") w189] -> w164
                      tunnel: w162 -> [_ w188]
                      tunnel: [string[][] [] ("Speed Data") w187] -> w161
                      tunnel: [w177 w186] -> w160
                      tunnel: w157 -> [w177 w185]
                      tunnel: [0 ("Actual number of speed values") w183] -> w155
                      tunnel: w151 -> [_ w182]
                      tunnel: w150 -> [_ w180]
                      frame False {
                      }
                      frame True {
                        n97 = call "Viewer speed UI interface.vi"("Caller"=enum16{"Viewer", "Exporter"}."Viewer", "Funct data structure"=w180, "Function"=enum16{"Initialise", "Update"}."Initialise", "error in (no error)"=w185, "Gobal frame number in Timelapse data/master video (1 based)"=w182, "Number of Frames"=w188, "Speed Data folder path+dummy filename"=w190) -> ("error out"=w186:errorcluster, "Speed Data"=w187:string[][], "Actual number of speed values"=w183:i32, "Speed waveform graph data"=w189:dbl[])  [unwired: 1 in]
                      }
                    }
                    "Speed Data" <- w161
                    "Actual number \nof speed points" <- w155
                    n98 = local write "Image"(w163) -> ()
                    n99 = call <vilib>:"Clear Errors.vi"("error in (no error)"=w152) -> ()  [unwired: 5 in, 2 out]
                    n100 = local write "VL Image Array"(w144) -> ()
                    n101 = property on="Speed Data" class="Arr (strict)"("Index Values"=u32[] [0]) -> ()  [unwired: 2 in, 2 out]
                    n102 = local write "Speed Graph"(w164) -> ()
                    n103 = call <vilib>:"Clear Errors.vi"("error in (no error)"=w160) -> ("error out"=w158:errorcluster)  [unwired: 5 in, 1 out]
                    n104 = call "Attempt to close binary refs.vi"("error in (no error)"=w158) -> ("error out"=w159:errorcluster)  [unwired: 10 in]
                    n105 = case shown="True" w145 {
                      tunnel: w159 -> [w169 w173]
                      tunnel: [T15 {"Vid 1"=refnum, "Vid 2"=refnum, "Vid 3"=refnum, "Vid 4"=refnum, "Vid1 Rel time (ms)"=0, "Vid2 Rel time (ms)"=0, "Vid3 Rel time (ms)"=0, "Vid4 Rel time (ms)"=0} ("Cam videos cluster") w172] -> w156
                      tunnel: [w169 w171] -> w153
                      tunnel: w150 -> [_ w170]
                      frame False {
                      }
                      frame True {
                        n106 = call "Read one frame from each bin file.vi"("Funct data structure"=w170, "error in (no error)"=w173, "Master video's frame number (unity-based)"=0 ("Frame number"), "Get/set"=Get-Set-Clear_Control."Set" ("GEt set .bin refs")) -> ("Error out"=w171:errorcluster, "Cam videos cluster"=w172:T15)  [unwired: 6 in]
                      }
                    }
                    n107 = flat-sequence {
                      tunnel: w156 -> [_]
                      frame #0 {
                        n108 = call <vilib>:"Unset Busy.vi"() -> ()  [unwired: 11 in, 1 out]
                      }
                    }
                    n109 = local write "Cams"(w156) -> ()
                    n110 = call <vilib>:"Clear Errors.vi"("error in (no error)"=w153) -> ()  [unwired: 5 in, 2 out]
                  }
                }
              }
            }
          }
          frame "Back to start" {
            w198 = 0 ("Scrollbar")
            n111 = call "Set Play-Stop buttons.vi"("Function"=Select_Play-Stop_button_to_show."Show Play button") -> ()  [unwired: 10 in, 1 out]
            n112 = global read "gl_Time series viewer globals.vi" "Start/End frame"() -> (w200:T36)
            n113 = property on="Scrollbar" class="Scroll (strict)"("Val(Sgnl)"=w198) -> ()  [unwired: 2 in, 2 out]
            n114 = Unbundle By Name(w200) -> ("Start Frame No"=w199:i32)
            n115 = local write "Slider at frame #"(w198) -> ()
            n116 = call "AVI-Reinitialise viewer on error.vi"("error in (no error)"=w203, "Queue in"=w201) -> ("error out"=w202:errorcluster)  [unwired: 9 in]
          }
          frame "Playback" {
            n117 = global read "gl_Time series viewer globals.vi" "# of Frames"() -> (w208:u32)
            n118 = while {
              tunnel: w214 -> [w234]
              tunnel: [w235] -> w210
              shift-right: [w232] -> w213
              shift-left: w212 -> [w223]
              tunnel: w208 -> [w227]
              tunnel: [0.0 ("Expected speed points")] -> w207
              tunnel: w205 -> [w216]
              stop <- w220 stop-if-true
              w217 = TRUE  # Funct acq data
              # "AVI Playback Loop"
              n119 = local write "Slider at frame #"(w223) -> ()
              n120 = local write "Scrollbar"(w223) -> ()
              n121 = local read "Stop"() -> (w228:bool)
              n122 = global read "General Globals.vi" "Stop application"() -> (w218:bool)
              n123 = call "Vol-Play.vi"("State"=w216, "Cycle number (in)"=w223, "error in (no error)"=w234, "Stop button pressed"=w228, "Number of Frames"=w227) -> ("error out"=w235:errorcluster, "Cycle number (out)"=w232:i32, "Speed data waveform graph"=→"Speed Graph":dbl[], "I mage ref out"=→"Image":T1, "Playback stopped"=w221:bool, "Image Array"=→"VL Image Array":T1[])  [unwired: 1 in]
              n124 = call "Read one frame from each bin file.vi"("Funct data structure"=w217, "Master video's frame number (unity-based)"=w223, "Get/set"=Get-Set-Clear_Control."Get" ("GEt set .bin refs")) -> ("Error out"=w219:errorcluster, "Cam videos cluster"=→"Cams":T15)  [unwired: 7 in]
              n125 = call "AVI playback timing control.vi"() -> ("Actual frame rate (fps)"=→"Actual frame rate (fps)":dbl, "Frame rate set OR original (fps)"=→"Frame rate set (fps)":dbl, "Original frame rate (fps)"=→"Original frame rate (fps)":dbl)  [unwired: 8 in, 1 out]
              n126 = Compound Arithmetic op=OR(w218, w219, w221) -> (w220:bool)
            }
            n127 = local write "Actual frame rate (fps)"(w207) -> ()
            n128 = call "AVI-Reinitialise viewer on error.vi"("error in (no error)"=w210, "Queue in"=w209) -> ("error out"=w211:errorcluster)  [unwired: 9 in]
            n129 = global read "General Globals.vi" "Stop application"() -> (w206:bool)
          }
          frame "Scroll bar event", "Speed cursor event" {
            n130 = case shown="No Error" w241 {
              selector: w241 -> [_ w264]
              tunnel: [w256 w263] -> w242
              tunnel: [w253 w264] -> w238
              tunnel: w240 -> [_ w263]
              tunnel: w236 -> [w252 _]
              frame No Error {
                w248 = TRUE  # Funct acq data
                # "Error handled internally"
                n131 = local read "Scrollbar"() -> (w255:i32)
                "Slider at frame #" <- w255
                n132 = global read "gl_Time series viewer globals.vi" "# of Frames"() -> (w246:u32)
                n133 = local read "Stop"() -> (w245:bool)
                n134 = call "Vol-Play.vi"("State"=w252, "Cycle number (in)"=w255, "Stop button pressed"=w245, "Number of Frames"=w246) -> ("error out"=w254:errorcluster, "Speed data waveform graph"=w247:dbl[], "I mage ref out"=w244:T1, "Image Array"=w243:T1[])  [unwired: 2 in, 2 out]
                n135 = call "Read one frame from each bin file.vi"("Funct data structure"=w248, "Master video's frame number (unity-based)"=w255, "Get/set"=Get-Set-Clear_Control."Get" ("GEt set .bin refs")) -> ("Error out"=w249:errorcluster, "Cam videos cluster"=w251:T15)  [unwired: 7 in]
                n136 = local write "VL Image Array"(w243) -> ()
                n137 = local write "Image"(w244) -> ()
                n138 = local write "Speed Graph"(w247) -> ()
                n139 = local write "Cams"(w251) -> ()
                n140 = call <vilib>:"Clear Errors.vi"("error in (no error)"=w249) -> ()  [unwired: 5 in, 2 out]
                n141 = flat-sequence {
                  tunnel: [w260] -> w256
                  tunnel: w255 -> [w258]
                  tunnel: [w257] -> w253
                  tunnel: w254 -> [w257]
                  frame #0 {
                    n142 = local write "Stop"(FALSE ("Stop")) -> ()
                    n143 = In Range and Coerce(upper limit=2147483647, x=w258, lower limit=1) -> (coerced(x)=w260:i32)  [unwired: 1 out]
                  }
                }
              }
              frame Error {
              }
            }
            n144 = call "AVI-Reinitialise viewer on error.vi"("error in (no error)"=w238, "Queue in"=w237) -> ("error out"=w239:errorcluster)  [unwired: 9 in]
          }
          frame "Exit" {
            n145 = local read "Stop"() -> (w268:bool)
            n146 = case shown="True" w268 {
              frame False {
              }
              frame True {
                n147 = local write "Stop"(FALSE ("Stop")) -> ()
              }
            }
          }
        }
      }
      frame True {
        # "Timeout"
        n148 = global read "General Globals.vi" "Stop application"() -> (w270:bool)
      }
    }
  }
  "Stop (ind)" <- w23
  n149 = while {
    tunnel: w20 -> [_]
    tunnel: [w273] -> w9
    stop <- w273 stop-if-true
    # "8-BIT VIDEO EXPORT LOOP"
    n150 = local read "Export vid"() -> (w274:bool)
    n151 = case shown="False" w274 {
      frame False {
        n152 = Wait Until Next ms Multiple(millisecond multiple=u32 200) -> ()  [unwired: 1 out]
      }
      frame True {
        w278 = FALSE ("Export")
        n153 = call <vilib>:"Set Busy.vi"() -> ("error out"=w277:errorcluster)  [unwired: 10 in, 1 out]
        n154 = local write "Export vid"(w278) -> ()
        n155 = flat-sequence {
          tunnel: w278 -> [_]
          tunnel: w277 -> [w282]
          tunnel: [w282] -> w276
          frame #0 {
            w279 = TRUE  # Funct data
            n156 = call "8-bit video export-setup.vi"("Funct data?"=w279) -> ("output cluster"=w281:T38, "cancelled"=w280:bool)  [unwired: 8 in, 1 out]
            n157 = case shown="False" w280 {
              tunnel: w281 -> [w283 _]
              frame False {
                n158 = disable-structure shown="Enabled" {
                  disable-tunnel: w283 -> [w284 w285]
                  frame Disabled {
                    n159 = call "Window-Exporting 8bit videos.vi"("Input cluster"=w284) -> ()  [unwired: 11 in]
                  }
                  frame Enabled {
                    n160 = call "Functional acq video generator.vi"("Input cluster"=w285) -> ()  [unwired: 11 in]
                  }
                }
              }
              frame True {
              }
            }
          }
        }
        n161 = call <vilib>:"Unset Busy.vi"("error in (no error)"=w276) -> ()  [unwired: 10 in, 1 out]
      }
    }
    n162 = local read "Stop (ind)"() -> (w273:bool)
  }
  n163 = while {
    shift-right: [w292] -> _
    shift-left: w26 -> [w291]
    tunnel: w37 -> [w290]
    shift-right: [w289] -> _
    shift-left: _ -> [w288]
    tunnel: [w287] -> w12
    tunnel: w13 -> [w286]
    tunnel: [w286] -> w14
    stop <- w293 stop-if-true
    # "EVENT HANDLING LOOP"
    n164 = event shown="[0] Timeout" {
      selector: _ -> [_ _ _ _ _ _ _ _ _ _ _ _ _ _ _ _ _ _ _]
      dyn-events: _ -> [_ _ _ _ _ _ _ _ _ _ _ _ _ _ _ _ _ _ _]
      timeout: 250 -> [_ _ _ _ _ _ _ _ _ _ _ _ _ _ _ _ _ _ _]
      tunnel: [w295 w301 _ _ _ _ _ _ _ _ _ _ _ _ _ _ _ _ w437] -> w293
      tunnel: [w299 w304 w315 w319 w333 w339 w347 w360 w374 w379 w384 w392 w397 w402 w405 w413 w415 w432 w439] -> w292
      tunnel: w291 -> [w299 w304 w315 w321 w333 w339 w347 w362 w374 w379 w384 w392 w397 w402 w405 w413 w417 w432 w439]
      tunnel: w290 -> [_ w302 _ w320 _ w340 _ w361 _ w378 _ _ _ w399 _ _ w421 _ w438]
      tunnel: [w298 w300 w316 w318 w332 w342 w346 w351 w370 w376 w380 FALSE FALSE w398 w404 w412 w418 w431 w436] -> w289
      tunnel: w288 -> [w298 w300 w316 w318 w332 w342 w346 w351 w370 w376 _ w391 _ w398 w404 w412 w418 w431 w436]
      tunnel: [w296 _ _ _ _ _ _ _ _ _ _ _ _ _ _ _ _ _ w435] -> w287
      tunnel: w286 -> [w297 _ _ _ _ _ _ _ _ _ _ _ _ _ _ _ _ _ w434]
      event Timeout {
        n165 = event-data() -> ()  [unwired: 1 in, 1 out]
        n166 = call "Funct Viewer-Bring to front.vi"() -> ()  [unwired: 12 in]
        n167 = global read "General Globals.vi" "Stop application"() -> (w295:bool)
        n168 = property class="VI"(reference=w297) -> ("FP.State"=w296:T39)  [unwired: 1 in, 2 out]
      }
      event Menu Selection (User) {
        n169 = event-data() -> ("ItemTag"=w303:string)  [unwired: 1 in]
        n170 = case shown="\"Close\"" w303 {
          tunnel: w302 -> [_ w305 _ _ w310 _ _ _]
          tunnel: [_ _ _ _ w309 _ _ _] -> w301
          frame Default {
          }
          frame "Load dataset" {
            n171 = call "Time series viewer-Event handler-Load dataset.vi"("queue"=w305) -> ()  [unwired: 11 in]
          }
          frame "Playback speed..." {
            n172 = call "Window-Playback speed entry.vi"() -> ("Frame rate set (fps)"=w306:dbl)  [unwired: 10 in, 1 out]
            n173 = local write "Frame rate set (fps)"(w306) -> ()
          }
          frame "Original speed (x1)" {
            n174 = flat-sequence {
              frame #0 {
                n175 = global write "gl_Time series viewer globals.vi" "Use manual FPS?"(FALSE ("Use manual FPS?")) -> ()
              }
              frame #1 {
                n176 = call "AVI playback timing control.vi"() -> ("Frame rate set OR original (fps)"=w308:dbl)  [unwired: 8 in, 3 out]
                n177 = local write "Frame rate set (fps)"(w308) -> ()
              }
            }
          }
          frame "Close" {
            n178 = call "Time series viewer-Event handler-Exit.vi"("Queue in"=w310) -> ("Exit"=w309:bool)  [unwired: 10 in]
            n179 = case shown="True" w309 {
              frame False {
              }
              frame True {
                n180 = local write "Stop"(TRUE ("Stop")) -> ()
              }
            }
          }
          frame "Export snippet" {
            "Export snippet" <- TRUE
          }
          frame "Export 8-bit video" {
            "Export vid" <- TRUE
          }
          frame "Export TIFF series" {
            "Export images" <- TRUE
          }
        }
      }
      event "Scrollbar", "Speed Graph": Shortcut Menu Selection (User) {
        n181 = event-data() -> ("ItemTag"=w317:string)  [unwired: 1 in]
        n182 = call "Time series viewer-Shortcut menu handler.vi"("ItemTag"=w317) -> ()  [unwired: 11 in]
      }
      event "Scrollbar": Value Change {
        n183 = event-data() -> ()  [unwired: 1 in, 1 out]
        n184 = disable-structure shown="Enabled" {
          disable-tunnel: w321 -> [w324 _]
          disable-tunnel: w320 -> [w323 w325]
          disable-tunnel: [w322 _] -> w319
          frame Enabled {
            n185 = call "Event case-Scrollbar value change.vi"("Tick count in"=w324, "Queue in"=w323) -> ("Tick count"=w322:u32)  [unwired: 8 in, 1 out]
          }
          frame Disabled {
            n186 = Lossy Enqueue Element(queue=w325, element=Speed_Viewer_States_enum."Scroll bar event" ("States")) -> ()  [unwired: 1 in, 4 out]
          }
        }
      }
      event "Speed Graph": Shortcut Menu Activation? {
        n187 = event-data() -> ("MenuRef"=w329:refnum<k9>)  [unwired: 1 in]
        n188 = call "FGV_Speed graph behaviour-Main viewer.vi"("Function"=Get-Set-Clear_Control."Get") -> ("Speed graph behaviour"=w328:T40)  [unwired: 9 in, 1 out]
        n189 = case shown="\"Scrolling data\", Default" w328 {
          tunnel: [bool[] [FALSE, TRUE] bool[] [TRUE, FALSE]] -> w327
          frame "Scrolling data", Default {
          }
          frame "Scrolling cursor" {
          }
        }
        n190 = for {
          tunnel: string[] ["scrolling cursor", "scrolling data"] -> [w338] mode=indexing
          tunnel: w329 -> [w337]
          tunnel: w327 -> [w336] mode=indexing
          n191 = Set Menu Item Info(6:w336, 7:w338, 11:w337) -> ()  [unwired: 4 in, 2 out]
        }
        n192 = event-data() -> ()  [unwired: 2 in, 1 out]
      }
      event "Speed Graph": Cursor Move; "Speed Graph": Cursor Release {
        n193 = event-data() -> ("CursRef"=w341:refnum<vi>)  [unwired: 1 in]
        n194 = call "Event case-Speed graph cursor moved.vi"("queue in"=w340, "Cursor in"=w341) -> ()  [unwired: 9 in, 1 out]
      }
      event "Speed Graph": event type 3.0.x80000027 {
        n195 = event-data() -> ()  [unwired: 1 in, 1 out]
        n196 = call "FGV_Speed graph behaviour-Main viewer.vi"("Function"=Get-Set-Clear_Control."Get") -> ("Speed graph behaviour"=w344:T40)  [unwired: 9 in, 1 out]
        n197 = case shown="\"Scrolling data\", Default" w344 {
          tunnel: [TRUE FALSE] -> w343
          frame "Scrolling data", Default {
            # "Moving the speed data graph's cursor manually is \nprevented when the mode is \"Scrolling data\"."
          }
          frame "Scrolling cursor" {
            # "Moving the speed data graph's cursor manually is \nallowed when the mode is \"Scrolling cursor\"."
          }
        }
        n198 = event-data("Discard?"=w343) -> ()  [unwired: 1 in, 1 out]
      }
      event "Extraction Cursors": Value Change {
        # "Do not use the left cursor's change event"
        # "Sets the main slider to the value of the extraction cursor that was moved."
        n199 = event-data() -> ("OldVal"=w359:cluster{i32, i32}, "NewVal"=w352:cluster{i32, i32})  [unwired: 1 in]
        n200 = Not Equal?(x=w359, y=w352) -> (x != y?=w353:cluster{bool, bool})
        n201 = Unbundle(w353) -> (w350:bool)  [unwired: 1 out]
        n202 = Unbundle(w352) -> (w358:i32, w357:i32)
        n203 = Select(t=w357, s=w350, f=w358) -> (s? t:f=w354:i32)
        n204 = flat-sequence {
          tunnel: w361 -> [w365]
          tunnel: w362 -> [w366]
          tunnel: [w366] -> w356
          tunnel: [w365] -> w355
          tunnel: w354 -> [w364]
          tunnel: w350 -> [w363]
          tunnel: [w367] -> w360
          tunnel: w356 -> [w369]
          tunnel: w355 -> [w368]
          frame #0 {
            n205 = call "Sync scrollbars.vi"("Min cursor moved"=w363, "Scrollbar value"=w364) -> ()  [unwired: 9 in, 1 out]
          }
          frame #1 {
            n206 = call "Event case-Scrollbar value change.vi"("Tick count in"=w369, "Queue in"=w368) -> ("Tick count"=w367:u32)  [unwired: 8 in, 1 out]
          }
        }
      }
      event Value Change {
        n207 = event-data() -> ()  [unwired: 1 in, 1 out]
        n208 = call "Prepare image colour.vi"("Left Image Palette"="Colour") -> ("Color Palette"=w371:cluster{"Red":u8, "Green":u8, "Blue":u8}[], "Palette Type"=w372:u32)  [unwired: 8 in, 1 out]
        n209 = property on="Image" class="ImageControl"("Palette Type"=w372, "User Palette"=w371) -> ()  [unwired: 2 in, 2 out]
      }
      event "Experiment Path", "Number of rows to generate": Value Change {
        n210 = event-data() -> ()  [unwired: 1 in, 1 out]
        n211 = Enqueue Element At Opposite End(queue=w378, element=Speed_Viewer_States_enum."Initialise") -> ()  [unwired: 2 in, 3 out]
        n212 = local write "Stop"(TRUE ("Stop")) -> ()
      }
      event "Cams.Vid 1", "Cams.Vid 2", "Cams.Vid 3", "Cams.Vid 4": Mouse Down {
        # "http://zone.ni.com/reference/en-XX/help/371361K-01/lvhowto/drag_and_drop_programmatic_prepare/"
        # "Detects and registers when the mouse is clicked \nwithin the boundaries of a CamVid display. This allows to generate a \"Drag leave\" event for those displays (in a separate event case / Mouse leave case).\nThis is necessary because the Drag-Leave event does not work for this type of control."
        n213 = event-data() -> ("Button"=w381:u16, "Mods.Double Click"=w383:bool, "CtlRef"=w382:refnum<vi>)  [unwired: 1 in]
        n214 = case shown="True" w383 {
          tunnel: w381 -> [_ w386]
          tunnel: w382 -> [_ w388]
          frame False {
          }
          frame True {
            n215 = property class="ImageControl"(reference=w388) -> ("Label.Text"=w387:string)  [unwired: 1 in, 2 out]
            n216 = call "Open expanded image window.vi"("Button"=w386, "Image name"=w387) -> ()  [unwired: 10 in]
          }
        }
        n217 = case shown="1" w381 {
          tunnel: [_ TRUE] -> w380
          frame 0, Default {
          }
          frame 1 {
          }
        }
      }
      event "Cams.Vid 1", "Cams.Vid 2", "Cams.Vid 3", "Cams.Vid 4": Mouse Leave {
        n218 = event-data() -> ("CtlRef"=w389:refnum<vi>)  [unwired: 1 in]
        n219 = case shown="False" w391 {
          tunnel: w389 -> [_ w395]
          frame False {
          }
          frame True {
            n220 = property class="ImageControl"(reference=w395) -> ("Label.Text"=w393:string)  [unwired: 1 in, 2 out]
            n221 = call "Open expanded image window.vi"("Button"=u16 0, "Image name"=w393) -> ()  [unwired: 10 in]
          }
        }
      }
      event Mouse Up {
        n222 = event-data() -> ()  [unwired: 1 in, 1 out]
      }
      event "Back": Value Change {
        n223 = event-data() -> ()  [unwired: 1 in, 1 out]
        n224 = Enqueue Element At Opposite End(queue=w399, element=Speed_Viewer_States_enum."Back to start") -> ()  [unwired: 2 in, 3 out]
        n225 = local write "Stop"(TRUE ("Stop")) -> ()
      }
      event Value Change {
        n226 = event-data() -> ()  [unwired: 1 in, 1 out]
        n227 = global write "gl_Time series viewer globals.vi" "Intensity"("Intensity") -> ()
        n228 = call "16-bit display mapping.vi"() -> ()  [unwired: 11 in, 1 out]
      }
      event "Image Scrollbar": Value Change {
        n229 = event-data() -> ("NewVal"=w409:i32)  [unwired: 1 in]
        n230 = global read "gl_Time series viewer globals.vi" "Timelapse viewer refs"() -> (w411:T7)
        n231 = Unbundle By Name(w411) -> ("VL Image Array"=w410:refnum<vi>)
        n232 = Build Array(w409) -> (w408:i32[])
        n233 = To Unsigned Long Integer(number=w408) -> (unsigned 32bit integer=w407:u32[])
        n234 = property class="Arr (strict)"(reference=w410, "Index Values"=w407) -> (error out=w406:errorcluster)  [unwired: 1 in, 1 out]
        n235 = call "16-bit display mapping.vi"("error in (no error)"=w406) -> ()  [unwired: 10 in, 1 out]
      }
      event "Play": Value Change {
        n236 = event-data() -> ()  [unwired: 1 in, 1 out]
        n237 = flat-sequence {
          tunnel: w421 -> [w425]
          tunnel: [w425] -> w420
          tunnel: w417 -> [w422]
          tunnel: [w422] -> w416
          tunnel: w420 -> [w427]
          tunnel: [w427] -> w419
          tunnel: w416 -> [w426]
          tunnel: [w426] -> w414
          tunnel: w419 -> [w429]
          tunnel: [w428] -> w415
          tunnel: w414 -> [w428]
          frame #0 {
            n238 = local write "Stop"(FALSE ("Stop")) -> ()
            n239 = call "Set Play-Stop buttons.vi"("Function"=Select_Play-Stop_button_to_show."Show Stop button") -> ()  [unwired: 10 in, 1 out]
          }
          frame #1 {
            n240 = call "Set scrollbar at start.vi"("Queue in"=w427) -> ()  [unwired: 10 in, 1 out]
          }
          frame #2 {
            n241 = Enqueue Element(queue=w429, element=Speed_Viewer_States_enum."Playback" ("States")) -> ()  [unwired: 2 in, 3 out]
          }
        }
      }
      event "Stop": Value Change {
        n242 = event-data() -> ()  [unwired: 1 in, 1 out]
      }
      event Panel Close? {
        # "The panel close is always discarded here because it is closed conditionally in the yellow \"Save Windows Bounds\" vi."
        n243 = event-data() -> ()  [unwired: 1 in, 1 out]
        n244 = call "Time series viewer-Event handler-Exit.vi"("Queue in"=w438) -> ("Exit"=w437:bool)  [unwired: 10 in]
        n245 = case shown="True" w437 {
          frame False {
          }
          frame True {
            n246 = local write "Stop"(TRUE ("Stop")) -> ()
            n247 = global write "gl_Time series viewer globals.vi" "Close larger image windows"(TRUE ("Close larger image window")) -> ()
          }
        }
        n248 = property class="VI"(reference=w434) -> ("FP.State"=w435:T39)  [unwired: 1 in, 2 out]
        n249 = event-data("Discard?"=TRUE) -> ()  [unwired: 1 in, 1 out]
      }
    }
  }
  n250 = call "Funct Viewer-cleanup.vi"("error in (no error)"=w34, "I16 image ref"=w38) -> ("error out"=w11:errorcluster)  [unwired: 9 in]
  n251 = flat-sequence {
    tunnel: w16 -> [w445]
    tunnel: w14 -> [w443]
    tunnel: w12 -> [w444]
    tunnel: w11 -> [_]
    tunnel: w9 -> [_]
    frame #0 {
      n252 = disable-structure shown="Enabled" {
        disable-tunnel: [w446 FALSE ("Front Panel Window:Open")] -> w442
        frame Disabled {
          n253 = call <userlib>:"Detect_Application_Kind.vi"() -> ("Development System"=w447:bool)  [unwired: 9 in, 2 out]
          n254 = case shown="True" w447 {
            tunnel: [_ TRUE ("Front Panel Window:Open")] -> w446
            frame False {
            }
            frame True {
            }
          }
        }
        frame Enabled {
        }
      }
      n255 = call "Save_Windows_Bounds.vi"("FP.State"=w444, "Window Name (i.e. Key)"=w445, "Front Panel Window:Open"=w442, "Window VI's Ref"=w443) -> ()  [unwired: 7 in, 1 out]
    }
  }
